vi "WPI_CameraSet Image Sensor Property.vi"(8 "error in":errorcluster, 10 "Prop String":string, 11 "address":string="192.168.0.90") -> (0 "error out":errorcluster)   [LabVIEW 2017]
doc: "This software is licensed. Open the labview\\readme\\WPI Robotics Library Open Source License.txt file for more information."
panel:
  out "Complete Response":string
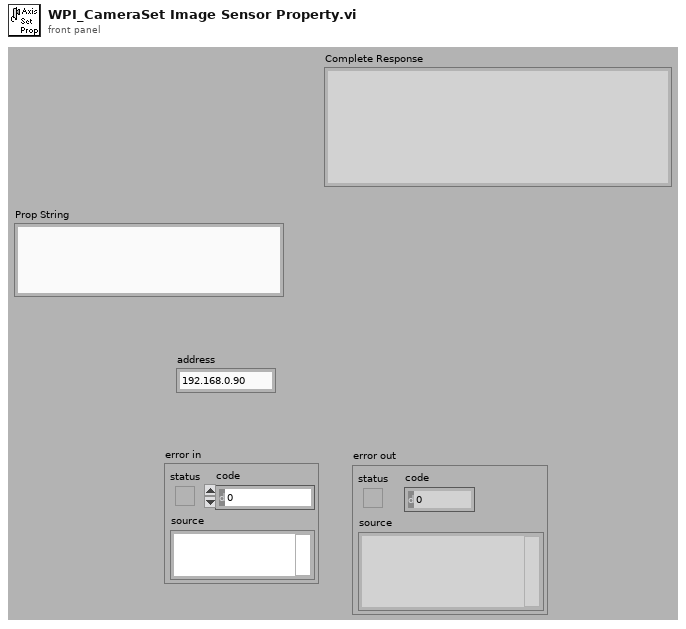
[diagram p1: front panel]
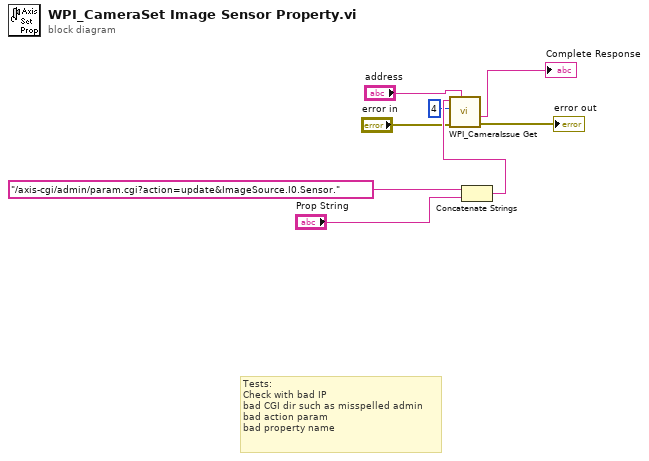
[diagram p0: block diagram]
diagram:
  # "Tests:\nCheck with bad IP\nbad CGI dir such as misspelled admin\nbad action param\nbad property name"
  n1 = Concatenate Strings("/axis-cgi/admin/param.cgi?action=update&ImageSource.I0.Sensor.", "Prop String") -> (w5:string)
  n2 = call <vilib>:"WPI_CameraIssue Get.vi"("address"="address", "error in (no error)"="error in", "Number of Lines Expected"=4, "Request"=w5) -> ("error out"=→"error out":errorcluster, "Complete Response"=→"Complete Response":string)  [unwired: 1 in, 5 out]
